vi "cam1analyse2.vi"(0 "W3":T1={"Global Rectangle"=[640, 450, 686, 504], "Contours"=[{"ID"=enum."External", "Type"=3, "Coordinates"=[640, 450, 686, 504]}]} {"Contours"."Type" items=["No Selection", "Point", "Line", "Rectangle", "Oval", "Polygon", "Freehand Region", "Annulus", "Unused2", "Unused3", "Broken Line", "Freehand Line", "Rotated Rectangle"]}, 7 "error in":errorcluster) -> (20 "W3":string[](array[string]), 27 "error out":errorcluster)   [LabVIEW 2019]
uses:
  <vilib>/vision/Classification.llb/IMAQ Classifier Read Options.ctl
  <vilib>/vision/NI_Vision_Development_Module.lvlib
panel:
  out "Coordinates":i32[](array[numeric])
  out "W3 chiffre":string
  out "R9 chiffre":string
  out "R8 chiffre":string
  out "R6 chiffre":string
  out "R3 chiffre":string
  out "B9 chiffre":string
  out "B8 chiffre":string
  out "B7 chiffre":string
  out "B6 chiffre":string
  out "B4 chiffre":string
  out "B3 chiffre":string
  out "B2 chiffre":string
  out "B1 chiffre":string
  out "W4 chiffre":string
  out "W6 chiffre":string
  out "W1 chiffre":string
  out "W2 chiffre":string
  in  "R9":T1={"Global Rectangle"=[0, 0, 1279, 959], "Contours"=[{"ID"=enum."External", "Type"=3, "Coordinates"=[0, 0, 1279, 959]}]} {"Contours"."Type" items=["No Selection", "Point", "Line", "Rectangle", "Oval", "Polygon", "Freehand Region", "Annulus", "Unused2", "Unused3", "Broken Line", "Freehand Line", "Rotated Rectangle"]}
  out "R9 2":string[](array[string])
  in  "R8":T1={"Global Rectangle"=[0, 0, 1279, 959], "Contours"=[{"ID"=enum."External", "Type"=3, "Coordinates"=[0, 0, 1279, 959]}]} {"Contours"."Type" items=["No Selection", "Point", "Line", "Rectangle", "Oval", "Polygon", "Freehand Region", "Annulus", "Unused2", "Unused3", "Broken Line", "Freehand Line", "Rotated Rectangle"]}
  out "R8 2":string[](array[string])
  in  "R6":T1={"Global Rectangle"=[0, 0, 1279, 959], "Contours"=[{"ID"=enum."External", "Type"=3, "Coordinates"=[0, 0, 1279, 959]}]} {"Contours"."Type" items=["No Selection", "Point", "Line", "Rectangle", "Oval", "Polygon", "Freehand Region", "Annulus", "Unused2", "Unused3", "Broken Line", "Freehand Line", "Rotated Rectangle"]}
  out "R6 2":string[](array[string])
  in  "R3":T1={"Global Rectangle"=[0, 0, 1279, 959], "Contours"=[{"ID"=enum."External", "Type"=3, "Coordinates"=[0, 0, 1279, 959]}]} {"Contours"."Type" items=["No Selection", "Point", "Line", "Rectangle", "Oval", "Polygon", "Freehand Region", "Annulus", "Unused2", "Unused3", "Broken Line", "Freehand Line", "Rotated Rectangle"]}
  out "R3 2":string[](array[string])
  in  "B9":T1={"Global Rectangle"=[0, 0, 1279, 959], "Contours"=[{"ID"=enum."External", "Type"=3, "Coordinates"=[0, 0, 1279, 959]}]} {"Contours"."Type" items=["No Selection", "Point", "Line", "Rectangle", "Oval", "Polygon", "Freehand Region", "Annulus", "Unused2", "Unused3", "Broken Line", "Freehand Line", "Rotated Rectangle"]}
  out "B9 2":string[](array[string])
  in  "B8":T1={"Global Rectangle"=[0, 0, 1279, 959], "Contours"=[{"ID"=enum."External", "Type"=3, "Coordinates"=[0, 0, 1279, 959]}]} {"Contours"."Type" items=["No Selection", "Point", "Line", "Rectangle", "Oval", "Polygon", "Freehand Region", "Annulus", "Unused2", "Unused3", "Broken Line", "Freehand Line", "Rotated Rectangle"]}
  out "B8 2":string[](array[string])
  in  "B7":T1={"Global Rectangle"=[0, 0, 1279, 959], "Contours"=[{"ID"=enum."External", "Type"=3, "Coordinates"=[0, 0, 1279, 959]}]} {"Contours"."Type" items=["No Selection", "Point", "Line", "Rectangle", "Oval", "Polygon", "Freehand Region", "Annulus", "Unused2", "Unused3", "Broken Line", "Freehand Line", "Rotated Rectangle"]}
  out "B7 2":string[](array[string])
  in  "B6":T1={"Global Rectangle"=[0, 0, 1279, 959], "Contours"=[{"ID"=enum."External", "Type"=3, "Coordinates"=[0, 0, 1279, 959]}]} {"Contours"."Type" items=["No Selection", "Point", "Line", "Rectangle", "Oval", "Polygon", "Freehand Region", "Annulus", "Unused2", "Unused3", "Broken Line", "Freehand Line", "Rotated Rectangle"]}
  out "B6 2":string[](array[string])
  in  "B4":T1={"Global Rectangle"=[0, 0, 1279, 959], "Contours"=[{"ID"=enum."External", "Type"=3, "Coordinates"=[0, 0, 1279, 959]}]} {"Contours"."Type" items=["No Selection", "Point", "Line", "Rectangle", "Oval", "Polygon", "Freehand Region", "Annulus", "Unused2", "Unused3", "Broken Line", "Freehand Line", "Rotated Rectangle"]}
  out "B4 2":string[](array[string])
  in  "B3":T1={"Global Rectangle"=[0, 0, 1279, 959], "Contours"=[{"ID"=enum."External", "Type"=3, "Coordinates"=[0, 0, 1279, 959]}]} {"Contours"."Type" items=["No Selection", "Point", "Line", "Rectangle", "Oval", "Polygon", "Freehand Region", "Annulus", "Unused2", "Unused3", "Broken Line", "Freehand Line", "Rotated Rectangle"]}
  out "B3 2":string[](array[string])
  in  "B2":T1={"Global Rectangle"=[0, 0, 1279, 959], "Contours"=[{"ID"=enum."External", "Type"=3, "Coordinates"=[0, 0, 1279, 959]}]} {"Contours"."Type" items=["No Selection", "Point", "Line", "Rectangle", "Oval", "Polygon", "Freehand Region", "Annulus", "Unused2", "Unused3", "Broken Line", "Freehand Line", "Rotated Rectangle"]}
  out "B2 2":string[](array[string])
  in  "B1":T1={"Global Rectangle"=[0, 0, 1279, 959], "Contours"=[{"ID"=enum."External", "Type"=3, "Coordinates"=[0, 0, 1279, 959]}]} {"Contours"."Type" items=["No Selection", "Point", "Line", "Rectangle", "Oval", "Polygon", "Freehand Region", "Annulus", "Unused2", "Unused3", "Broken Line", "Freehand Line", "Rotated Rectangle"]}
  out "B1 2":string[](array[string])
  in  "W4":T1={"Global Rectangle"=[0, 0, 1279, 959], "Contours"=[{"ID"=enum."External", "Type"=3, "Coordinates"=[0, 0, 1279, 959]}]} {"Contours"."Type" items=["No Selection", "Point", "Line", "Rectangle", "Oval", "Polygon", "Freehand Region", "Annulus", "Unused2", "Unused3", "Broken Line", "Freehand Line", "Rotated Rectangle"]}
  out "W4 2":string[](array[string])
  in  "W6":T1={"Global Rectangle"=[0, 0, 1279, 959], "Contours"=[{"ID"=enum."External", "Type"=3, "Coordinates"=[0, 0, 1279, 959]}]} {"Contours"."Type" items=["No Selection", "Point", "Line", "Rectangle", "Oval", "Polygon", "Freehand Region", "Annulus", "Unused2", "Unused3", "Broken Line", "Freehand Line", "Rotated Rectangle"]}
  out "W6 2":string[](array[string])
  in  "W1":T1={"Global Rectangle"=[0, 0, 1279, 959], "Contours"=[{"ID"=enum."External", "Type"=3, "Coordinates"=[0, 0, 1279, 959]}]} {"Contours"."Type" items=["No Selection", "Point", "Line", "Rectangle", "Oval", "Polygon", "Freehand Region", "Annulus", "Unused2", "Unused3", "Broken Line", "Freehand Line", "Rotated Rectangle"]}
  out "W1 2":string[](array[string])
  in  "W2 2":T1={"Global Rectangle"=[0, 0, 1279, 959], "Contours"=[{"ID"=enum."External", "Type"=3, "Coordinates"=[0, 0, 1279, 959]}]} {"Contours"."Type" items=["No Selection", "Point", "Line", "Rectangle", "Oval", "Polygon", "Freehand Region", "Annulus", "Unused2", "Unused3", "Broken Line", "Freehand Line", "Rotated Rectangle"]}
  out "W2 3":string[](array[string])
  out "Image Out":T2(plugin-control)
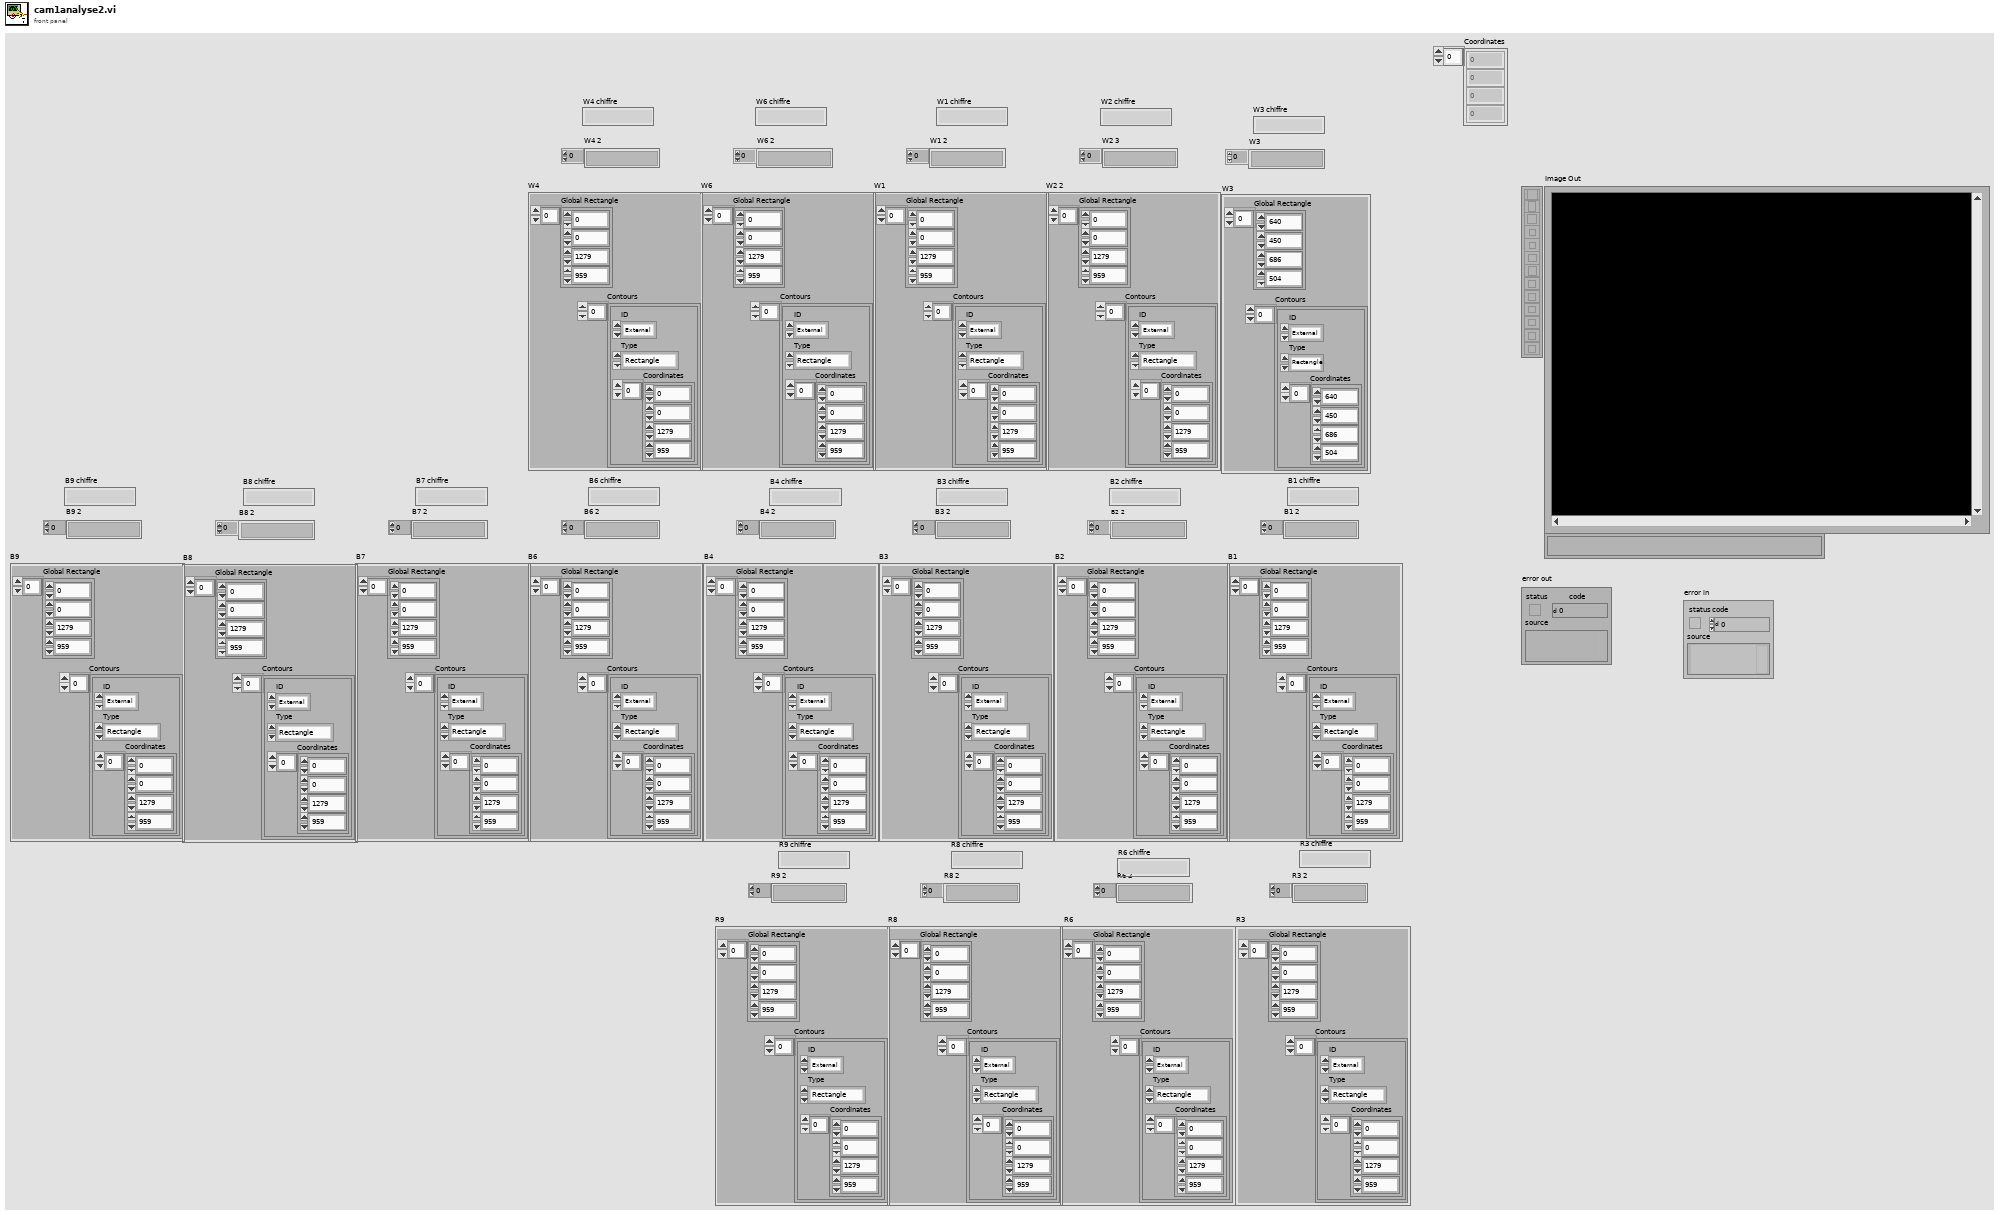
[diagram p1: front panel]
types:
  T1 = cluster{"Global Rectangle":i32[], "Contours":cluster{"ID":enum32{"External", "Internal"}, "Type":u32, "Coordinates":i32[]}[]}
  T2 = typedef "IMAQ Image.ctl" = refnum<image>
  T3 = typedef "IMAQ Classifier Read Options.ctl" = i32
  T4 = typedef "IMAQ Classifier Session.ctl" = refnum<k1>
  T5 = typedef "ROI Descriptor" = cluster{"Global Rectangle":i32[], "Contours":cluster{"ID":enum32{"External", "Internal"}, "Type":u32, "Coordinates":i32[]}[]}
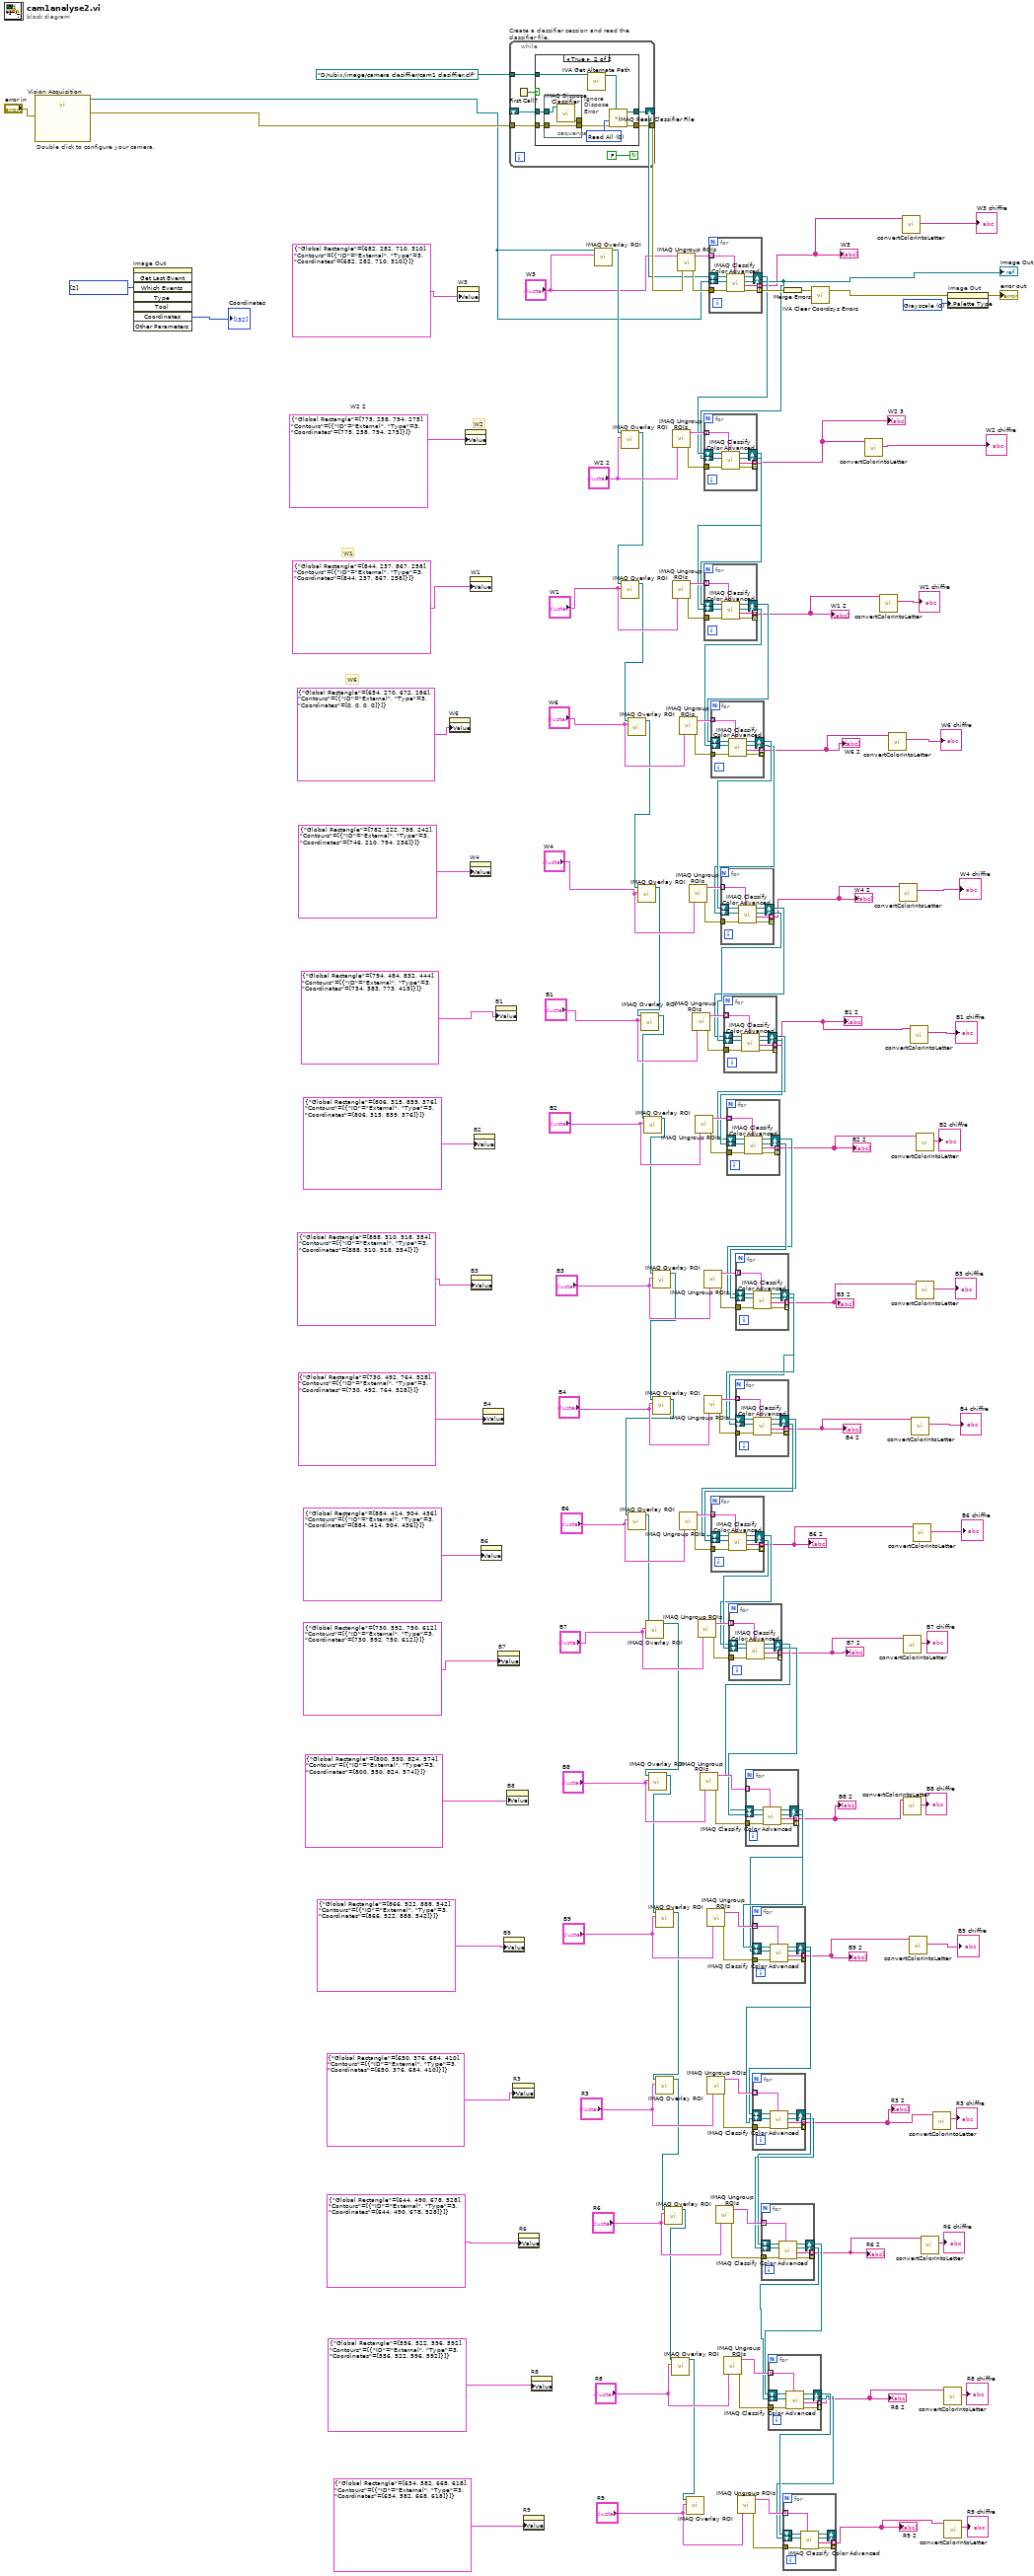
[diagram p0: block diagram]
diagram:
  w1 = i32[] [2] items=["No Event"=0, "Click Event"=1, "Draw Event"=2, "Size Event"=4, "Scroll Event"=5, "Double Click Event"=8] ("Which Events")
  w152 = u32 0 items=["Grayscale", "Binary", "Gradient", "Rainbow", "Temperature", "User Defined", "Binary 16 Bit", "Gradient 16 Bit", "Rainbow 16 Bit", "Temperature 16 Bit", "User Defined 16 Bit"] ("Palette Type")
  # "W2"
  # "W6"
  # "W1"
  # "Double click to configure your camera."
  n1 = call "Vision Acquisition"("error in"="error in") -> ("Image Out"=w5:T2, "error out"=w162:errorcluster)  [unwired: 24 in, 1 out]
  n2 = invoke on="Image Out" class="ImageControl" method="Get Last Event"("Which Events"=w1) -> ("Coordinates"=→"Coordinates":i32[])  [unwired: 7 in, 7 out]
  n3 = property on="W6" class="Clust (strict)"("Value"=T1 {"Global Rectangle"=[654, 270, 672, 286], "Contours"=[{"ID"=enum."External", "Type"=3, "Coordinates"=[0, 0, 0, 0]}]} ("ROI Descriptor (Color Classification 1)")) -> ()  [unwired: 2 in, 2 out]
  n4 = property on="W3" class="Clust (strict)"("Value"=T1 {"Global Rectangle"=[682, 282, 710, 310], "Contours"=[{"ID"=enum."External", "Type"=3, "Coordinates"=[682, 282, 710, 310]}]} ("ROI Descriptor (Color Classification 1)")) -> ()  [unwired: 2 in, 2 out]
  n5 = property on="W2 2" class="Clust (strict)"("Value"=T1 {"Global Rectangle"=[775, 258, 794, 275], "Contours"=[{"ID"=enum."External", "Type"=3, "Coordinates"=[775, 258, 794, 275]}]} ("ROI Descriptor (Color Classification 1)")) -> ()  [unwired: 2 in, 2 out]
  n6 = property on="W4" class="Clust (strict)"("Value"=T1 {"Global Rectangle"=[782, 222, 798, 242], "Contours"=[{"ID"=enum."External", "Type"=3, "Coordinates"=[746, 210, 794, 236]}]} ("ROI Descriptor (Color Classification 1)")) -> ()  [unwired: 2 in, 2 out]
  n7 = property on="W1" class="Clust (strict)"("Value"=T1 {"Global Rectangle"=[844, 237, 867, 258], "Contours"=[{"ID"=enum."External", "Type"=3, "Coordinates"=[844, 237, 867, 258]}]} ("ROI Descriptor (Color Classification 1)")) -> ()  [unwired: 2 in, 2 out]
  n8 = property on="B3" class="Clust (strict)"("Value"=T1 {"Global Rectangle"=[888, 310, 918, 354], "Contours"=[{"ID"=enum."External", "Type"=3, "Coordinates"=[888, 310, 918, 354]}]} ("ROI Descriptor (Color Classification 1)")) -> ()  [unwired: 2 in, 2 out]
  n9 = property on="B2" class="Clust (strict)"("Value"=T1 {"Global Rectangle"=[806, 315, 859, 376], "Contours"=[{"ID"=enum."External", "Type"=3, "Coordinates"=[806, 315, 859, 376]}]} ("ROI Descriptor (Color Classification 1)")) -> ()  [unwired: 2 in, 2 out]
  n10 = property on="B6" class="Clust (strict)"("Value"=T1 {"Global Rectangle"=[884, 414, 904, 436], "Contours"=[{"ID"=enum."External", "Type"=3, "Coordinates"=[884, 414, 904, 436]}]} ("ROI Descriptor (Color Classification 1)")) -> ()  [unwired: 2 in, 2 out]
  n11 = property on="B4" class="Clust (strict)"("Value"=T1 {"Global Rectangle"=[730, 492, 764, 528], "Contours"=[{"ID"=enum."External", "Type"=3, "Coordinates"=[730, 492, 764, 528]}]} ("ROI Descriptor (Color Classification 1)")) -> ()  [unwired: 2 in, 2 out]
  n12 = property on="B1" class="Clust (strict)"("Value"=T1 {"Global Rectangle"=[794, 484, 832, 444], "Contours"=[{"ID"=enum."External", "Type"=3, "Coordinates"=[734, 383, 773, 419]}]} ("ROI Descriptor (Color Classification 1)")) -> ()  [unwired: 2 in, 2 out]
  n13 = property on="B7" class="Clust (strict)"("Value"=T1 {"Global Rectangle"=[730, 592, 750, 612], "Contours"=[{"ID"=enum."External", "Type"=3, "Coordinates"=[730, 592, 750, 612]}]} ("ROI Descriptor (Color Classification 1)")) -> ()  [unwired: 2 in, 2 out]
  n14 = property on="B9" class="Clust (strict)"("Value"=T1 {"Global Rectangle"=[866, 522, 888, 542], "Contours"=[{"ID"=enum."External", "Type"=3, "Coordinates"=[866, 522, 888, 542]}]} ("ROI Descriptor (Color Classification 1)")) -> ()  [unwired: 2 in, 2 out]
  n15 = property on="B8" class="Clust (strict)"("Value"=T1 {"Global Rectangle"=[800, 550, 824, 574], "Contours"=[{"ID"=enum."External", "Type"=3, "Coordinates"=[800, 550, 824, 574]}]} ("ROI Descriptor (Color Classification 1)")) -> ()  [unwired: 2 in, 2 out]
  n16 = while "Create a classifier session and read the classifier file." {
    shift-right: [w170] -> w154
    shift-left: _ -> [w169]
    tunnel: w162 -> [w167]
    tunnel: [w166] -> w160
    tunnel: path "D:/rubix/image/camera clasiffier/cam1 clasiffier.clf" ("File Path") -> [w165]
    stop <- FALSE continue-if-true
    n17 = First Call?() -> (First Call?: T/F=w164:bool)
    n18 = case shown="True" w164 {
      tunnel: [w172 w179] -> w170
      tunnel: w169 -> [w172 w177]
      tunnel: w167 -> [w171 w176]
      tunnel: [w171 w178] -> w166
      tunnel: w165 -> [_ w174]
      frame False {
      }
      frame True {
        w180 = T3 0 items=["Read All", "Add Samples, Do Not Change Options", "Read Options, Do Not Add Samples"] ("Read Options")
        # "Ignore Dispose Error"
        n19 = stacked-sequence {
          tunnel: w177 -> [w183]
          tunnel: w176 -> [w182]
          tunnel: [w182] -> w175
          tunnel: [w181] -> _
          frame #0 {
            n20 = call "IMAQ Dispose Classifier"("Classifier Session"=w183) -> ("error out"=w181:errorcluster)  [unwired: 1 in, 9 out]
          }
        }
        n21 = call <vilib>:"IVA Get Alternate Path.vi"("Path In"=w174) -> ("Path Out"=w173:path)  [unwired: 10 out]
        n22 = call "IMAQ Read Classifier File"("File Path"=w173, "error in (no error)"=w175, "Read Options"=w180) -> ("error out"=w178:errorcluster, "Classifier Session"=w179:T4)  [unwired: 1 in, 6 out]
      }
    }
  }
  n23 = property on="R3" class="Clust (strict)"("Value"=T1 {"Global Rectangle"=[650, 376, 684, 410], "Contours"=[{"ID"=enum."External", "Type"=3, "Coordinates"=[650, 376, 684, 410]}]} ("ROI Descriptor (Color Classification 1)")) -> ()  [unwired: 2 in, 2 out]
  n24 = property on="R6" class="Clust (strict)"("Value"=T1 {"Global Rectangle"=[644, 490, 678, 528], "Contours"=[{"ID"=enum."External", "Type"=3, "Coordinates"=[644, 490, 678, 528]}]} ("ROI Descriptor (Color Classification 1)")) -> ()  [unwired: 2 in, 2 out]
  n25 = property on="R9" class="Clust (strict)"("Value"=T1 {"Global Rectangle"=[634, 582, 668, 618], "Contours"=[{"ID"=enum."External", "Type"=3, "Coordinates"=[634, 582, 668, 618]}]} ("ROI Descriptor (Color Classification 1)")) -> ()  [unwired: 2 in, 2 out]
  n26 = property on="R8" class="Clust (strict)"("Value"=T1 {"Global Rectangle"=[556, 522, 596, 592], "Contours"=[{"ID"=enum."External", "Type"=3, "Coordinates"=[556, 522, 596, 592]}]} ("ROI Descriptor (Color Classification 1)")) -> ()  [unwired: 2 in, 2 out]
  n27 = call "IMAQ Overlay ROI"("ROI Descriptor"="W3", "Image"=w5) -> ("Image Out"=w10:T2)  [unwired: 8 in, 1 out]
  n28 = call "IMAQ Overlay ROI"("ROI Descriptor"="W2 2", "Image"=w10) -> ("Image Out"=w145:T2)  [unwired: 8 in, 1 out]
  n29 = call "IMAQ Overlay ROI"("ROI Descriptor"="W1", "Image"=w145) -> ("Image Out"=w137:T2)  [unwired: 8 in, 1 out]
  n30 = call "IMAQ Overlay ROI"("ROI Descriptor"="W6", "Image"=w137) -> ("Image Out"=w129:T2)  [unwired: 8 in, 1 out]
  n31 = call "IMAQ Overlay ROI"("ROI Descriptor"="W4", "Image"=w129) -> ("Image Out"=w122:T2)  [unwired: 8 in, 1 out]
  n32 = call "IMAQ Overlay ROI"("ROI Descriptor"="B1", "Image"=w122) -> ("Image Out"=w117:T2)  [unwired: 8 in, 1 out]
  n33 = call "IMAQ Overlay ROI"("ROI Descriptor"="B2", "Image"=w117) -> ("Image Out"=w110:T2)  [unwired: 8 in, 1 out]
  n34 = call "IMAQ Overlay ROI"("ROI Descriptor"="B3", "Image"=w110) -> ("Image Out"=w100:T2)  [unwired: 8 in, 1 out]
  n35 = call "IMAQ Overlay ROI"("ROI Descriptor"="B4", "Image"=w100) -> ("Image Out"=w96:T2)  [unwired: 8 in, 1 out]
  n36 = call "IMAQ Overlay ROI"("ROI Descriptor"="B6", "Image"=w96) -> ("Image Out"=w87:T2)  [unwired: 8 in, 1 out]
  n37 = call "IMAQ Overlay ROI"("ROI Descriptor"="B7", "Image"=w87) -> ("Image Out"=w82:T2)  [unwired: 8 in, 1 out]
  n38 = call "IMAQ Overlay ROI"("ROI Descriptor"="B8", "Image"=w82) -> ("Image Out"=w75:T2)  [unwired: 8 in, 1 out]
  n39 = call "IMAQ Overlay ROI"("ROI Descriptor"="B9", "Image"=w75) -> ("Image Out"=w68:T2)  [unwired: 8 in, 1 out]
  n40 = call "IMAQ Overlay ROI"("ROI Descriptor"="R3", "Image"=w68) -> ("Image Out"=w61:T2)  [unwired: 8 in, 1 out]
  n41 = call "IMAQ Overlay ROI"("ROI Descriptor"="R6", "Image"=w61) -> ("Image Out"=w54:T2)  [unwired: 8 in, 1 out]
  n42 = call "IMAQ Overlay ROI"("ROI Descriptor"="R8", "Image"=w54) -> ("Image Out"=w47:T2)  [unwired: 8 in, 1 out]
  n43 = call "IMAQ Ungroup ROIs"("ROI Descriptor"="W2 2") -> ("error out"=w151:errorcluster, "ROI Descriptors out"=w150:T5[])  [unwired: 1 in, 2 out]
  n44 = call "IMAQ Ungroup ROIs"("ROI Descriptor"="W1") -> ("error out"=w147:errorcluster, "ROI Descriptors out"=w146:T5[])  [unwired: 1 in, 2 out]
  n45 = call "IMAQ Ungroup ROIs"("error in (no error)"=w160, "ROI Descriptor"="W3") -> ("error out"=w159:errorcluster, "ROI Descriptors out"=w158:T5[])  [unwired: 2 out]
  n46 = call "IMAQ Ungroup ROIs"("ROI Descriptor"="W6") -> ("error out"=w140:errorcluster, "ROI Descriptors out"=w139:T5[])  [unwired: 1 in, 2 out]
  n47 = call "IMAQ Ungroup ROIs"("ROI Descriptor"="B6") -> ("error out"=w99:errorcluster, "ROI Descriptors out"=w98:T5[])  [unwired: 1 in, 2 out]
  n48 = call "IMAQ Overlay ROI"("ROI Descriptor"="R9", "Image"=w47) -> ()  [unwired: 8 in, 2 out]
  n49 = call "IMAQ Ungroup ROIs"("ROI Descriptor"="W4") -> ("error out"=w133:errorcluster, "ROI Descriptors out"=w132:T5[])  [unwired: 1 in, 2 out]
  n50 = call "IMAQ Ungroup ROIs"("ROI Descriptor"="B1") -> ("error out"=w126:errorcluster, "ROI Descriptors out"=w125:T5[])  [unwired: 1 in, 2 out]
  n51 = call "IMAQ Ungroup ROIs"("ROI Descriptor"="B2") -> ("error out"=w120:errorcluster, "ROI Descriptors out"=w119:T5[])  [unwired: 1 in, 2 out]
  n52 = call "IMAQ Ungroup ROIs"("ROI Descriptor"="B7") -> ("error out"=w92:errorcluster, "ROI Descriptors out"=w91:T5[])  [unwired: 1 in, 2 out]
  n53 = call "IMAQ Ungroup ROIs"("ROI Descriptor"="B8") -> ("error out"=w85:errorcluster, "ROI Descriptors out"=w84:T5[])  [unwired: 1 in, 2 out]
  n54 = call "IMAQ Ungroup ROIs"("ROI Descriptor"="B4") -> ("error out"=w106:errorcluster, "ROI Descriptors out"=w105:T5[])  [unwired: 1 in, 2 out]
  n55 = call "IMAQ Ungroup ROIs"("ROI Descriptor"="B3") -> ("error out"=w113:errorcluster, "ROI Descriptors out"=w112:T5[])  [unwired: 1 in, 2 out]
  n56 = call "IMAQ Ungroup ROIs"("ROI Descriptor"="B9") -> ("error out"=w78:errorcluster, "ROI Descriptors out"=w77:T5[])  [unwired: 1 in, 2 out]
  n57 = call "IMAQ Ungroup ROIs"("ROI Descriptor"="R3") -> ("error out"=w71:errorcluster, "ROI Descriptors out"=w70:T5[])  [unwired: 1 in, 2 out]
  n58 = for {
    tunnel: [w191] -> w8 mode=indexing
    tunnel: [w190] -> w157 mode=indexing
    tunnel: w159 -> [w188]
    tunnel: w158 -> [w187] mode=indexing
    shift-right: [w185] -> w11
    shift-left: w5 -> [w186]
    shift-right: [w184] -> w12
    shift-left: w154 -> [w189]
    n59 = call "IMAQ Classify Color Advanced"("ROI Descriptor"=w187, "error in (no error)"=w188, "Image"=w186, "Classifier Session"=w189) -> ("error out"=w190:errorcluster, "Class"=w191:string, "Image (dup)"=w185:T2, "Classifier Session (dup)"=w184:T4)  [unwired: 4 out]
  }
  "W3" <- w8
  "Image Out" <- w11
  n60 = for {
    tunnel: [w199] -> w4 mode=indexing
    tunnel: [w198] -> _ mode=indexing
    tunnel: w151 -> [w196]
    tunnel: w150 -> [w195] mode=indexing
    shift-right: [w193] -> w143
    shift-left: w11 -> [w194]
    shift-right: [w192] -> w144
    shift-left: w12 -> [w197]
    n61 = call "IMAQ Classify Color Advanced"("ROI Descriptor"=w195, "error in (no error)"=w196, "Image"=w194, "Classifier Session"=w197) -> ("error out"=w198:errorcluster, "Class"=w199:string, "Image (dup)"=w193:T2, "Classifier Session (dup)"=w192:T4)  [unwired: 4 out]
  }
  "W2 3" <- w4
  n62 = for {
    tunnel: [w207] -> w42 mode=indexing
    tunnel: [w206] -> _ mode=indexing
    tunnel: w147 -> [w204]
    tunnel: w146 -> [w203] mode=indexing
    shift-right: [w201] -> w136
    shift-left: w143 -> [w202]
    shift-right: [w200] -> w135
    shift-left: w144 -> [w205]
    n63 = call "IMAQ Classify Color Advanced"("ROI Descriptor"=w203, "error in (no error)"=w204, "Image"=w202, "Classifier Session"=w205) -> ("error out"=w206:errorcluster, "Class"=w207:string, "Image (dup)"=w201:T2, "Classifier Session (dup)"=w200:T4)  [unwired: 4 out]
  }
  "W1 2" <- w42
  n64 = for {
    tunnel: [w215] -> w41 mode=indexing
    tunnel: [w214] -> _ mode=indexing
    tunnel: w140 -> [w212]
    tunnel: w139 -> [w211] mode=indexing
    shift-right: [w209] -> w130
    shift-left: w136 -> [w210]
    shift-right: [w208] -> w131
    shift-left: w135 -> [w213]
    n65 = call "IMAQ Classify Color Advanced"("ROI Descriptor"=w211, "error in (no error)"=w212, "Image"=w210, "Classifier Session"=w213) -> ("error out"=w214:errorcluster, "Class"=w215:string, "Image (dup)"=w209:T2, "Classifier Session (dup)"=w208:T4)  [unwired: 4 out]
  }
  "W6 2" <- w41
  n66 = call "IMAQ Ungroup ROIs"("ROI Descriptor"="R6") -> ("error out"=w64:errorcluster, "ROI Descriptors out"=w63:T5[])  [unwired: 1 in, 2 out]
  n67 = for {
    tunnel: [w223] -> w40 mode=indexing
    tunnel: [w222] -> _ mode=indexing
    tunnel: w133 -> [w220]
    tunnel: w132 -> [w219] mode=indexing
    shift-right: [w217] -> w124
    shift-left: w130 -> [w218]
    shift-right: [w216] -> w123
    shift-left: w131 -> [w221]
    n68 = call "IMAQ Classify Color Advanced"("ROI Descriptor"=w219, "error in (no error)"=w220, "Image"=w218, "Classifier Session"=w221) -> ("error out"=w222:errorcluster, "Class"=w223:string, "Image (dup)"=w217:T2, "Classifier Session (dup)"=w216:T4)  [unwired: 4 out]
  }
  "W4 2" <- w40
  n69 = call "IMAQ Ungroup ROIs"("ROI Descriptor"="R8") -> ("error out"=w57:errorcluster, "ROI Descriptors out"=w56:T5[])  [unwired: 1 in, 2 out]
  n70 = for {
    tunnel: [w231] -> w39 mode=indexing
    tunnel: [w230] -> _ mode=indexing
    tunnel: w126 -> [w228]
    tunnel: w125 -> [w227] mode=indexing
    shift-right: [w225] -> w116
    shift-left: w124 -> [w226]
    shift-right: [w224] -> w115
    shift-left: w123 -> [w229]
    n71 = call "IMAQ Classify Color Advanced"("ROI Descriptor"=w227, "error in (no error)"=w228, "Image"=w226, "Classifier Session"=w229) -> ("error out"=w230:errorcluster, "Class"=w231:string, "Image (dup)"=w225:T2, "Classifier Session (dup)"=w224:T4)  [unwired: 4 out]
  }
  "B1 2" <- w39
  n72 = for {
    tunnel: [w239] -> w38 mode=indexing
    tunnel: [w238] -> _ mode=indexing
    tunnel: w120 -> [w236]
    tunnel: w119 -> [w235] mode=indexing
    shift-right: [w233] -> w109
    shift-left: w116 -> [w234]
    shift-right: [w232] -> w108
    shift-left: w115 -> [w237]
    n73 = call "IMAQ Classify Color Advanced"("ROI Descriptor"=w235, "error in (no error)"=w236, "Image"=w234, "Classifier Session"=w237) -> ("error out"=w238:errorcluster, "Class"=w239:string, "Image (dup)"=w233:T2, "Classifier Session (dup)"=w232:T4)  [unwired: 4 out]
  }
  "B2 2" <- w38
  n74 = for {
    tunnel: [w247] -> w37 mode=indexing
    tunnel: [w246] -> _ mode=indexing
    tunnel: w113 -> [w244]
    tunnel: w112 -> [w243] mode=indexing
    shift-right: [w241] -> w103
    shift-left: w109 -> [w242]
    shift-right: [w240] -> w104
    shift-left: w108 -> [w245]
    n75 = call "IMAQ Classify Color Advanced"("ROI Descriptor"=w243, "error in (no error)"=w244, "Image"=w242, "Classifier Session"=w245) -> ("error out"=w246:errorcluster, "Class"=w247:string, "Image (dup)"=w241:T2, "Classifier Session (dup)"=w240:T4)  [unwired: 4 out]
  }
  "B3 2" <- w37
  n76 = for {
    tunnel: [w255] -> w36 mode=indexing
    tunnel: [w254] -> _ mode=indexing
    tunnel: w106 -> [w252]
    tunnel: w105 -> [w251] mode=indexing
    shift-right: [w249] -> w95
    shift-left: w103 -> [w250]
    shift-right: [w248] -> w94
    shift-left: w104 -> [w253]
    n77 = call "IMAQ Classify Color Advanced"("ROI Descriptor"=w251, "error in (no error)"=w252, "Image"=w250, "Classifier Session"=w253) -> ("error out"=w254:errorcluster, "Class"=w255:string, "Image (dup)"=w249:T2, "Classifier Session (dup)"=w248:T4)  [unwired: 4 out]
  }
  "B4 2" <- w36
  n78 = for {
    tunnel: [w263] -> w35 mode=indexing
    tunnel: [w262] -> _ mode=indexing
    tunnel: w99 -> [w260]
    tunnel: w98 -> [w259] mode=indexing
    shift-right: [w257] -> w90
    shift-left: w95 -> [w258]
    shift-right: [w256] -> w89
    shift-left: w94 -> [w261]
    n79 = call "IMAQ Classify Color Advanced"("ROI Descriptor"=w259, "error in (no error)"=w260, "Image"=w258, "Classifier Session"=w261) -> ("error out"=w262:errorcluster, "Class"=w263:string, "Image (dup)"=w257:T2, "Classifier Session (dup)"=w256:T4)  [unwired: 4 out]
  }
  "B6 2" <- w35
  n80 = for {
    tunnel: [w271] -> w34 mode=indexing
    tunnel: [w270] -> _ mode=indexing
    tunnel: w92 -> [w268]
    tunnel: w91 -> [w267] mode=indexing
    shift-right: [w265] -> w81
    shift-left: w90 -> [w266]
    shift-right: [w264] -> w80
    shift-left: w89 -> [w269]
    n81 = call "IMAQ Classify Color Advanced"("ROI Descriptor"=w267, "error in (no error)"=w268, "Image"=w266, "Classifier Session"=w269) -> ("error out"=w270:errorcluster, "Class"=w271:string, "Image (dup)"=w265:T2, "Classifier Session (dup)"=w264:T4)  [unwired: 4 out]
  }
  "B7 2" <- w34
  n82 = call "IMAQ Ungroup ROIs"("ROI Descriptor"="R9") -> ("error out"=w50:errorcluster, "ROI Descriptors out"=w49:T5[])  [unwired: 1 in, 2 out]
  n83 = for {
    tunnel: [w279] -> w33 mode=indexing
    tunnel: [w278] -> _ mode=indexing
    tunnel: w85 -> [w276]
    tunnel: w84 -> [w275] mode=indexing
    shift-right: [w273] -> w73
    shift-left: w81 -> [w274]
    shift-right: [w272] -> w74
    shift-left: w80 -> [w277]
    n84 = call "IMAQ Classify Color Advanced"("ROI Descriptor"=w275, "error in (no error)"=w276, "Image"=w274, "Classifier Session"=w277) -> ("error out"=w278:errorcluster, "Class"=w279:string, "Image (dup)"=w273:T2, "Classifier Session (dup)"=w272:T4)  [unwired: 4 out]
  }
  "B8 2" <- w33
  n85 = for {
    tunnel: [w287] -> w32 mode=indexing
    tunnel: [w286] -> _ mode=indexing
    tunnel: w78 -> [w284]
    tunnel: w77 -> [w283] mode=indexing
    shift-right: [w281] -> w66
    shift-left: w73 -> [w282]
    shift-right: [w280] -> w67
    shift-left: w74 -> [w285]
    n86 = call "IMAQ Classify Color Advanced"("ROI Descriptor"=w283, "error in (no error)"=w284, "Image"=w282, "Classifier Session"=w285) -> ("error out"=w286:errorcluster, "Class"=w287:string, "Image (dup)"=w281:T2, "Classifier Session (dup)"=w280:T4)  [unwired: 4 out]
  }
  "B9 2" <- w32
  n87 = for {
    tunnel: [w295] -> w31 mode=indexing
    tunnel: [w294] -> _ mode=indexing
    tunnel: w71 -> [w292]
    tunnel: w70 -> [w291] mode=indexing
    shift-right: [w289] -> w59
    shift-left: w66 -> [w290]
    shift-right: [w288] -> w60
    shift-left: w67 -> [w293]
    n88 = call "IMAQ Classify Color Advanced"("ROI Descriptor"=w291, "error in (no error)"=w292, "Image"=w290, "Classifier Session"=w293) -> ("error out"=w294:errorcluster, "Class"=w295:string, "Image (dup)"=w289:T2, "Classifier Session (dup)"=w288:T4)  [unwired: 4 out]
  }
  "R3 2" <- w31
  n89 = for {
    tunnel: [w303] -> w30 mode=indexing
    tunnel: [w302] -> _ mode=indexing
    tunnel: w64 -> [w300]
    tunnel: w63 -> [w299] mode=indexing
    shift-right: [w297] -> w53
    shift-left: w59 -> [w298]
    shift-right: [w296] -> w52
    shift-left: w60 -> [w301]
    n90 = call "IMAQ Classify Color Advanced"("ROI Descriptor"=w299, "error in (no error)"=w300, "Image"=w298, "Classifier Session"=w301) -> ("error out"=w302:errorcluster, "Class"=w303:string, "Image (dup)"=w297:T2, "Classifier Session (dup)"=w296:T4)  [unwired: 4 out]
  }
  "R6 2" <- w30
  n91 = for {
    tunnel: [w311] -> w29 mode=indexing
    tunnel: [w310] -> _ mode=indexing
    tunnel: w57 -> [w308]
    tunnel: w56 -> [w307] mode=indexing
    shift-right: [w305] -> w45
    shift-left: w53 -> [w306]
    shift-right: [w304] -> w46
    shift-left: w52 -> [w309]
    n92 = call "IMAQ Classify Color Advanced"("ROI Descriptor"=w307, "error in (no error)"=w308, "Image"=w306, "Classifier Session"=w309) -> ("error out"=w310:errorcluster, "Class"=w311:string, "Image (dup)"=w305:T2, "Classifier Session (dup)"=w304:T4)  [unwired: 4 out]
  }
  "R8 2" <- w29
  n93 = for {
    tunnel: [w319] -> w28 mode=indexing
    tunnel: [w318] -> _ mode=indexing
    tunnel: w50 -> [w316]
    tunnel: w49 -> [w315] mode=indexing
    shift-right: [w313] -> _
    shift-left: w45 -> [w314]
    shift-right: [w312] -> _
    shift-left: w46 -> [w317]
    n94 = call "IMAQ Classify Color Advanced"("ROI Descriptor"=w315, "error in (no error)"=w316, "Image"=w314, "Classifier Session"=w317) -> ("error out"=w318:errorcluster, "Class"=w319:string, "Image (dup)"=w313:T2, "Classifier Session (dup)"=w312:T4)  [unwired: 4 out]
  }
  "R9 2" <- w28
  n95 = Merge Errors(w157) -> (w156:errorcluster)
  n96 = call <vilib>:"IVA Clear Coordsys Errors.vi"("error in (no error)"=w156) -> ("error out"=w155:errorcluster)  [unwired: 10 in]
  n97 = call "convertColorIntoLetter.vi"("Array"=w4) -> ("String"=→"W2 chiffre":string)  [unwired: 10 in]
  n98 = call "convertColorIntoLetter.vi"("Array"=w42) -> ("String"=→"W1 chiffre":string)  [unwired: 10 in]
  n99 = call "convertColorIntoLetter.vi"("Array"=w41) -> ("String"=→"W6 chiffre":string)  [unwired: 10 in]
  n100 = call "convertColorIntoLetter.vi"("Array"=w40) -> ("String"=→"W4 chiffre":string)  [unwired: 10 in]
  n101 = call "convertColorIntoLetter.vi"("Array"=w8) -> ("String"=→"W3 chiffre":string)  [unwired: 10 in]
  n102 = call "convertColorIntoLetter.vi"("Array"=w33) -> ("String"=→"B8 chiffre":string)  [unwired: 10 in]
  n103 = call "convertColorIntoLetter.vi"("Array"=w34) -> ("String"=→"B7 chiffre":string)  [unwired: 10 in]
  n104 = call "convertColorIntoLetter.vi"("Array"=w32) -> ("String"=→"B9 chiffre":string)  [unwired: 10 in]
  n105 = call "convertColorIntoLetter.vi"("Array"=w39) -> ("String"=→"B1 chiffre":string)  [unwired: 10 in]
  n106 = call "convertColorIntoLetter.vi"("Array"=w36) -> ("String"=→"B4 chiffre":string)  [unwired: 10 in]
  n107 = call "convertColorIntoLetter.vi"("Array"=w35) -> ("String"=→"B6 chiffre":string)  [unwired: 10 in]
  n108 = call "convertColorIntoLetter.vi"("Array"=w38) -> ("String"=→"B2 chiffre":string)  [unwired: 10 in]
  n109 = call "convertColorIntoLetter.vi"("Array"=w37) -> ("String"=→"B3 chiffre":string)  [unwired: 10 in]
  n110 = call "convertColorIntoLetter.vi"("Array"=w30) -> ("String"=→"R6 chiffre":string)  [unwired: 10 in]
  n111 = call "convertColorIntoLetter.vi"("Array"=w31) -> ("String"=→"R3 chiffre":string)  [unwired: 10 in]
  n112 = call "convertColorIntoLetter.vi"("Array"=w29) -> ("String"=→"R8 chiffre":string)  [unwired: 10 in]
  n113 = call "convertColorIntoLetter.vi"("Array"=w28) -> ("String"=→"R9 chiffre":string)  [unwired: 10 in]
  n114 = property on="Image Out" class="ImageControl"(error in=w155, "Palette:Palette Type"=w152) -> (error out=→"error out":errorcluster)  [unwired: 1 in, 1 out]
